vi "Tegam4040 -- Test OpenClose.vi"() -> ()   [LabVIEW 2010]
panel:
  out "error out":errorcluster
  out "Dac Value":u16 format="%x"
  in  "Timeout (5000 msecs)":i32=5000
  in  "Reset Device?":bool
  in  "VISA Resource In":refnum<visa-resource-name>
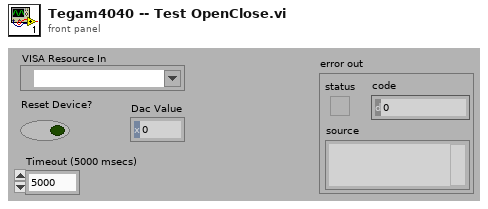
[diagram p1: front panel]
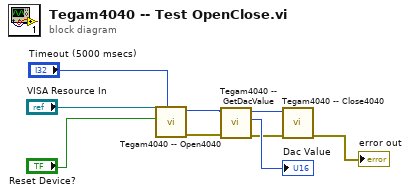
[diagram p0: block diagram]
diagram:
  n1 = call "Tegam4040 -- Open4040.vi"("Timeout (5000 msecs)"="Timeout (5000 msecs)", "Reset Device?"="Reset Device?", "VISA Resource In"="VISA Resource In") -> ("error out"=w6:errorcluster, "Instrument Session Handle"=w5:u32)  [unwired: 7 in]
  n2 = call "Tegam4040 -- GetDacValue.vi"("error in (no error)"=w6, "Instrument Session Handle In"=w5) -> ("error out"=w3:errorcluster, "Dac Value"=→"Dac Value":u16, "Instrument Session Handle Out (dupl)"=w2:u32)  [unwired: 7 in]
  n3 = call "Tegam4040 -- Close4040.vi"("error in (no error)"=w3, "Instrument Session Handle"=w2) -> ("error out"=→"error out":errorcluster)  [unwired: 9 in]
